vi "Configure Waveform Modulation (FSK).vi"(6 "FSK Rate (1000 Hz)":dbl=1000.0, 8 "error in (no error)":errorcluster, 9 "Hop Frequency (2000 Hz)":dbl=2000.0, 10 "Waveform Generator Number (1: Waveform Generator 1)":i32(ring)=1 items=["Waveform Generator 1"=1], 11 "VISA resource name":refnum<visa-resource-name>) -> (0 "error out":errorcluster, 3 "VISA resource name out":refnum<visa-resource-name>)   [LabVIEW 2015, in "Agilent 2000 3000 X-Series.lvlib"]
doc: "Configures the waveform modulation FSK."
uses:
  <instrlib>/Agilent 2000 3000 X-Series/Agilent 2000 3000 X-Series.lvlib
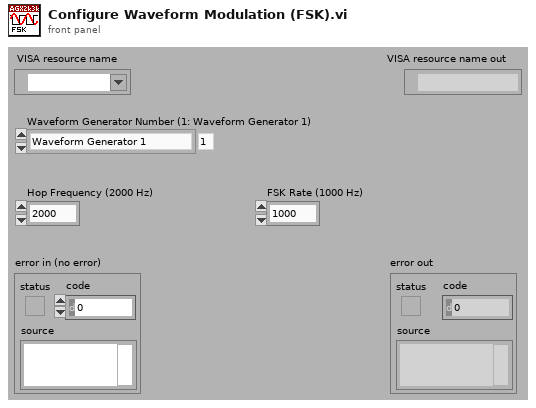
[diagram p1: front panel]
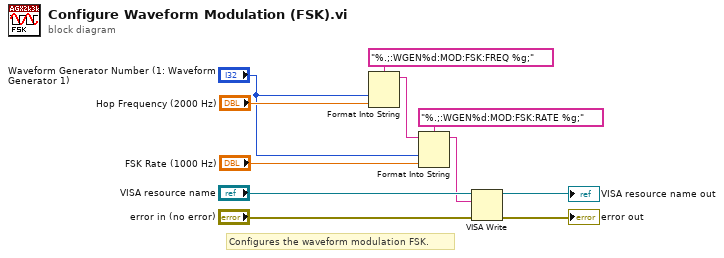
[diagram p0: block diagram]
diagram:
  # "Configures the waveform modulation FSK."
  n1 = Format Into String(format string="%.;:WGEN%d:MOD:FSK:FREQ %g;", "Waveform Generator Number (1: Waveform Generator 1)", "Hop Frequency (2000 Hz)") -> (resulting string=w5:string)  [unwired: 2 in, 1 out]
  n2 = Format Into String(format string="%.;:WGEN%d:MOD:FSK:RATE %g;", initial string=w5, "Waveform Generator Number (1: Waveform Generator 1)", "FSK Rate (1000 Hz)") -> (resulting string=w1:string)  [unwired: 1 in, 1 out]
  n3 = VISA Write(VISA resource name="VISA resource name", write buffer=w1, error in (no error)="error in (no error)") -> (VISA resource name out=→"VISA resource name out":refnum<visa-resource-name>, error out=→"error out":errorcluster)  [unwired: 1 out]
